vi "Flatten.vi"(4 "T_Out":u64, 6 "T0":u64, 8 "error in (no error)":errorcluster, 10 "Data":T1 {"payload" format="%x"; "identifier" format="%x"}, 11 "CIFTag in":refnum<class "CIFFifoCAN.lvclass">) -> (0 "error out":errorcluster, 3 "CIFTag out":refnum<class "CIFFifoCAN.lvclass">)   [LabVIEW 2021, in "CIFFifoCAN.lvclass"]
uses:
  CIFFifoCAN.lvclass
  CIFFIFO/CIFfifo.lvclass
  ChannelCommon/ChannelCommon.lvlib
  e2488641-f297-4923-bbd0-3c2628a14485.vi
  ChannelRegistrar/typedef/Datatype CAN.ctl
  ChannelRegistrar/ChannelRegistrar.lvlib
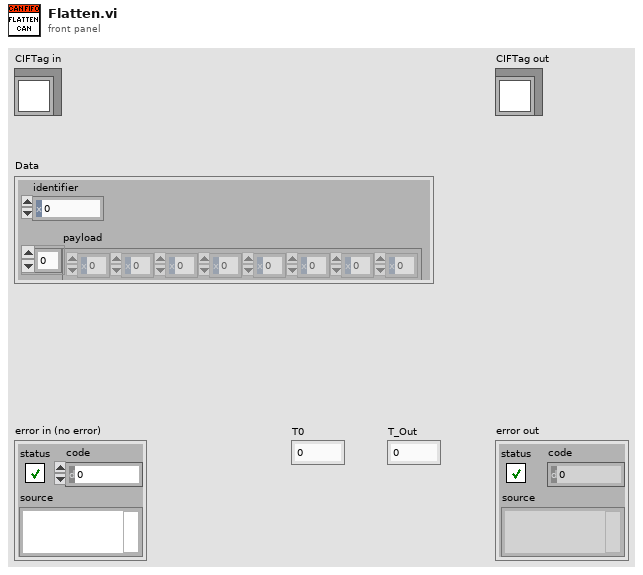
[diagram p1: front panel]
types:
  T1 = typedef "ChannelRegistrar.lvlib/Datatype CAN.ctl" = cluster{"payload":u8[], "identifier":u32}
  T2 = typedef "ChannelCommon.lvlib/FIFO Header.ctl" = cluster{"Length":u64, "T0":u64, "T_Out":u64, "T_Tx":u64, "Ctr":u64}
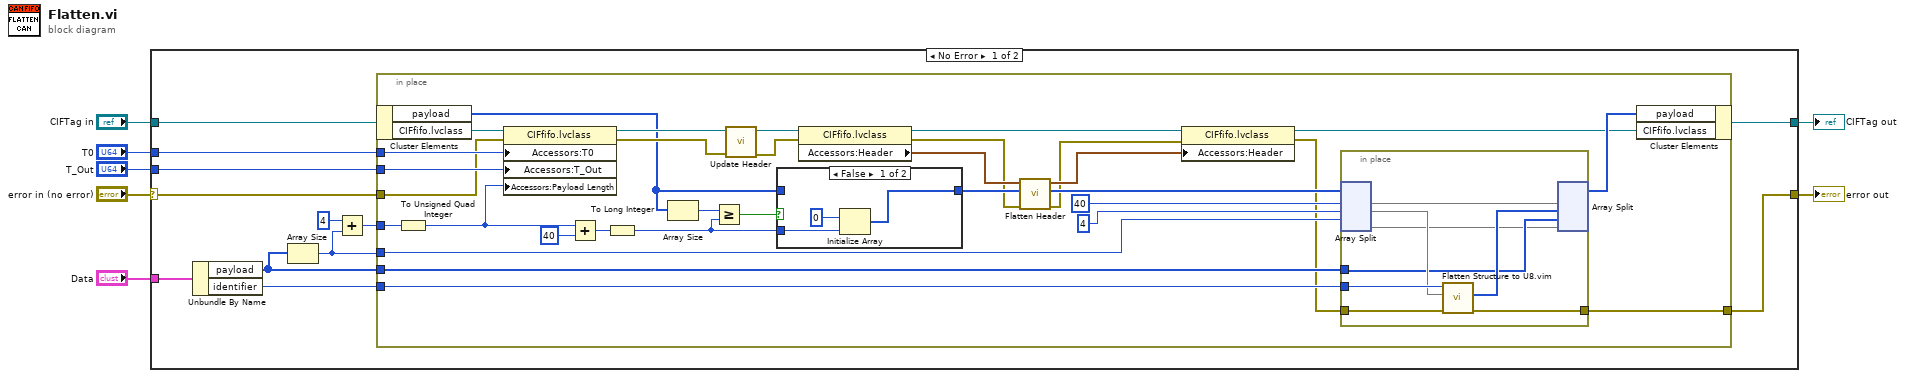
[diagram p0: block diagram]
diagram:
  n1 = case shown="No Error" "error in (no error)" {
    selector: "error in (no error)" -> [w17 w65]
    tunnel: [w9 w65] -> w6
    tunnel: [w8 w64] -> w4
    tunnel: "CIFTag in" -> [w16 w64]
    tunnel: "T_Out" -> [w19 _]
    tunnel: "T0" -> [w18 _]
    tunnel: "Data" -> [w15 _]
    frame No Error {
      n2 = Unbundle By Name(w15) -> ("payload"=w11:u8[], "identifier"=w12:u32)
      n3 = Array Size(array=w11) -> (size(s)=w10:i32)
      n4 = Add(x=4 ("y"), y=w10) -> (x+y=w13:i32)
      n5 = in-place {
        in-place-border: w19 -> [w48]
        in-place-border: w18 -> [w47]
        in-place-border: w17 -> [w46]
        in-place-border: w13 -> [w43]
        in-place-border: w12 -> [w31]
        in-place-border: w11 -> [w30]
        in-place-border: w10 -> [w29]
        in-place-border: [w25] -> w9
        n6 = in-place-cluster #1(w16) -> ("payload"=w37:u8[], "CIFfifo.lvclass"=w51:refnum<class "CIFfifo.lvclass">)
        n7 = To Unsigned Quad Integer(1:w43) -> (0:w41:u64)
        n8 = property class="CIFfifo.lvclass"(reference=w51, error in=w46, "Accessors:T0"=w47, "Accessors:T_Out"=w48, "Accessors:Payload Length"=w41) -> (reference out=w50:refnum<class "CIFfifo.lvclass">, error out=w49:errorcluster)
        n9 = Add(x=w41, y=u64 40) -> (x+y=w26:u64)
        n10 = To Long Integer(number=w26) -> (32bit integer=w28:i32)
        n11 = Array Size(array=w37) -> (size(s)=w39:i32)
        n12 = Greater Or Equal?(x=w39, y=w28) -> (x >= y?=w38:bool)
        n13 = call "Update Header.vi"("error in (no error)"=w49, "CIFFIFO in"=w50) -> ("error out"=w44:errorcluster, "CIFFIFO out"=w45:refnum<class "CIFfifo.lvclass">)  [unwired: 8 in]
        n14 = case shown="False" w38 {
          tunnel: w37 -> [_ w63]
          tunnel: [w60 w63] -> w36
          tunnel: w28 -> [w62 _]
          frame False {
            n15 = Initialize Array(u8 0, w62) -> (w60:u8[])
          }
          frame True {
          }
        }
        n16 = property class="CIFfifo.lvclass"(reference=w45, error in=w44) -> (reference out=w24:refnum<class "CIFfifo.lvclass">, error out=w35:errorcluster, "Accessors:Header"=w42:T2)
        n17 = call "Flatten Header.vi"("error in"=w35, "Flattened Data in"=w36, "Header in"=w42) -> ("error out"=w21:errorcluster, "Flattened Data out"=w34:u8[], "Header out"=w22:T2)  [unwired: 6 in]
        n18 = property class="CIFfifo.lvclass"(reference=w24, error in=w21, "Accessors:Header"=w22) -> (reference out=w23:refnum<class "CIFfifo.lvclass">, error out=w20:errorcluster)
        n19 = in-place {
          in-place-border: w31 -> [w58]
          in-place-border: w20 -> [w55]
          in-place-border: w30 -> [w54]
          in-place-border: [w52] -> w25
          n20 = in-place-split #2(w34, 40, 4, w29) -> (w59:u8[], w57:u8[], w53:u8[])  [unwired: 1 out]
          n21 = call "Flatten Structure to U8.vim"("error in"=w55, "Flattened Data in"=w57, "Data to Flatten in"=w58) -> ("error out"=w52:errorcluster, "Flattened Data out"=w56:u8[])  [unwired: 6 in, 1 out]
          n22 = in-place-split #2(w59, w56, w54, w53) -> (w27:u8[])  [unwired: 3 out]
        }
        n23 = in-place-cluster #1("payload"=w27, "CIFfifo.lvclass"=w23) -> (w8:refnum<class "CIFFifoCAN.lvclass">)
      }
    }
    frame Error {
    }
  }
  "error out" <- w6
  "CIFTag out" <- w4
